vi "全局变量.vi"() -> ()   [LabVIEW 2011]
panel:
  in  "Counts":i32
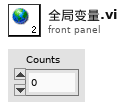
[diagram p1: front panel]
diagram:
